vi "Populate Ring Text [].vi"(8 "error in (no error)":errorcluster, 10 "Strings []":string[](array[string]), 11 "Ring in":refnum<vi>) -> (0 "error out":errorcluster)   [LabVIEW 2016, in "LV-Data.lvclass"]
uses:
  LV-Data.lvclass
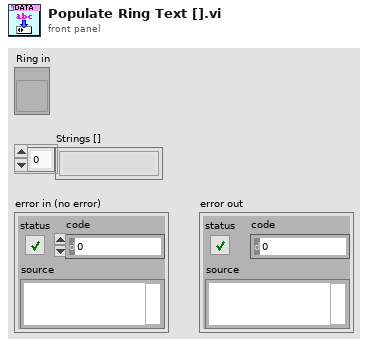
[diagram p1: front panel]
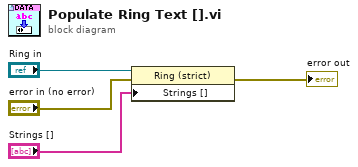
[diagram p0: block diagram]
diagram:
  n1 = property on="Property Node" class="Ring (strict)"(reference="Ring in", error in="error in (no error)", "Strings []"="Strings []") -> (error out=→"error out":errorcluster)  [unwired: 1 out]
